vi "FlatToRichGreeter_req.vi"(5 "OutputClusterType":T1, 11 "InputCluster":T2) -> (3 "OutputCluster":T1)   [LabVIEW 2019, in "Generated_server.lvlib"]
uses:
  Generated_server.lvlib
  Greeter_req_Flat.ctl
  Greeter_MessageA_Flat.ctl
  Greeter_req.ctl
  Greeter_req_req_oneof/Greeter_req_req_oneof.lvclass
  Greeter_req_req_oneof/Greeter_req_req_oneof.lvclass/Greeter_req_req_oneof.ctl
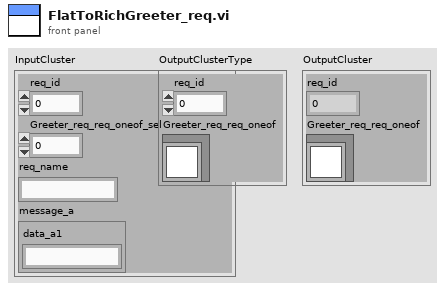
[diagram p1: front panel]
types:
  T1 = typedef "Generated_server.lvlib/Greeter_req.ctl" = cluster{"req_id":i32, "Greeter_req_req_oneof":refnum<class "Greeter_req_req_oneof.lvclass">}
  T2 = typedef "Generated_server.lvlib/Greeter_req_Flat.ctl" = cluster{"req_id":i32, "Greeter_req_req_oneof_selected_index":i32, "req_name":string, "message_a":T3}
  T3 = typedef "Generated_server.lvlib/Greeter_MessageA_Flat.ctl" = cluster{"data_a1":string}
  T4 = typedef "Generated_server.lvlib/Greeter_MessageA.ctl" = cluster{"data_a1":string}
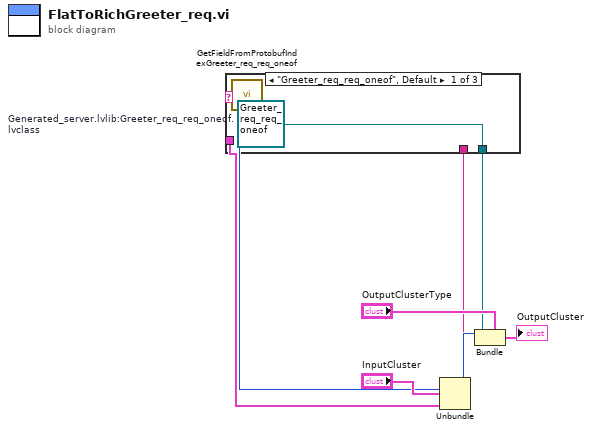
[diagram p0: block diagram]
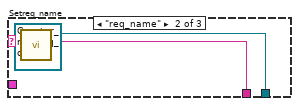
[diagram p2: hidden frame]
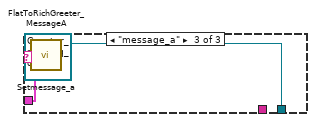
[diagram p3: hidden frame]
diagram:
  n1 = Unbundle "Unbundle"("InputCluster") -> ("req_id"=w6:i32, "Greeter_req_req_oneof_selected_index"=w5:i32, "req_name"=w2:string, "message_a"=w1:T3)
  n2 = call "GetFieldFromProtobufIndexGreeter_req_req_oneof.vi"("protobuf index"=w5) -> ("oneof field name"=w4:string)
  n3 = case "Greeter_req_req_oneof" shown="\"Greeter_req_req_oneof\", Default" w4 {
    tunnel: [w10 w12 w15] -> w3
    tunnel: w2 -> [_ w13 _]
    tunnel: w1 -> [_ _ w17]
    frame "Greeter_req_req_oneof", Default {
      w10 = refnum<class "Greeter_req_req_oneof.lvclass"> refnum  # Generated_server.lvlib:Greeter_req_req_oneof.lvclass
    }
    frame "req_name" {
      n4 = call "Setreq_name.vi"("Set_Val"=w13, "OneOfTemplate in"=refnum<class "Greeter_req_req_oneof.lvclass"> refnum) -> ("OneOfTemplate out"=w12:refnum<class "Greeter_req_req_oneof.lvclass">)  [unwired: 8 in, 1 out]
    }
    frame "message_a" {
      n5 = call "FlatToRichGreeter_MessageA.vi"("InputCluster"=w17) -> ("OutputCluster"=w16:T4)  [unwired: 10 in]
      n6 = call "Setmessage_a.vi"("Set_Val"=w16, "OneOfTemplate in"=refnum<class "Greeter_req_req_oneof.lvclass"> refnum) -> ("OneOfTemplate out"=w15:refnum<class "Greeter_req_req_oneof.lvclass">)  [unwired: 8 in, 1 out]
    }
  }
  n7 = Bundle "Bundle"(cluster="OutputClusterType", "req_id"=w6, "Greeter_req_req_oneof"=w3) -> (→"OutputCluster":T1)
